vi "Untitled 1.vi"() -> ()   [LabVIEW 2015]
uses:
  <vilib>/MakerHub/LINX/Public/Peripherals/Analog/Analog Read 1 Chan.vi
  <vilib>/MakerHub/LINX/Private/Local IO/LinxI2cWrite.vi
  <vilib>/MakerHub/LINX/Public/Utilities/Check Channel.vi
  <vilib>/MakerHub/LINX/Public/Peripherals/Analog/Analog Read N Chans.vi
  <vilib>/MakerHub/LINX/Private/Local IO/LinxAnalogRead.vi
  <vilib>/MakerHub/LINX/Public/Utilities/Open Serial.vi
  <vilib>/MakerHub/LINX/Private/Utilties/Generate Error.vi
  <vilib>/MakerHub/LINX/LMH-LINX.lvlib
panel:
  in  "DAC Output Voltage":sgl min=0 max=5 step=0.001
  in  "stop":bool
  out "Voltage 2":dbl
  out "Voltage":dbl
  in  "LED":refnum<visa-resource-name>="N/A"
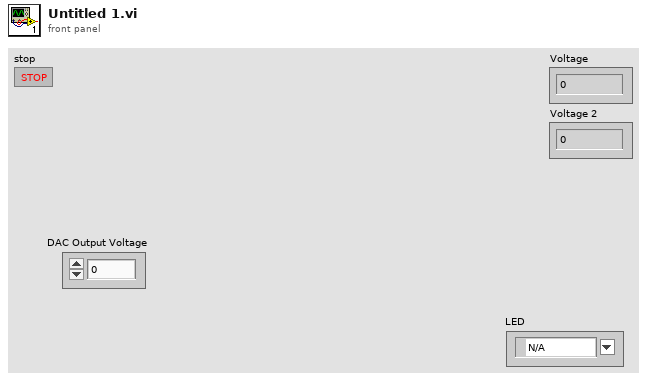
[diagram p1: front panel]
types:
  T1 = typedef "LMH-LINX.lvlib/LINX Ref.ctl" = cluster{"IO":T2, "Interface":T3, "LINX Device Config":T4}
  T2 = typedef "LMH-LINX.lvlib/Platform.ctl" = enum16{"Remote", "Local"}
  T3 = typedef "LMH-LINX.lvlib/Interface.ctl" = enum16{"Serial", "TCP"}
  T4 = typedef "LMH-LINX.lvlib/Device.lvlib/LINX Device Config.ctl" = cluster{"Interface":T3, "COM Port":refnum<visa-resource-name>, "TCP Configuration":T5, "Device Family":u8, "Device ID":u8, "Device Name":string, "TCP Ref":refnum<k5>, "Channels":T6}
  T5 = typedef "LMH-LINX.lvlib/Device.lvlib/TCP Config.ctl" = cluster{"IP Address":string, "Port":u16}
  T6 = typedef "LMH-LINX.lvlib/Channels.ctl" = cluster{"DI":u8[], "DO":u8[], "AI":u8[], "AO":u8[], "PWM":u8[], "QE":u8[], "UART":u8[], "I2C 2":u8[], "SPI":u8[], "CAN":u8[], "Servo":u8[], "AI Ref (V)":dbl, "AI Resolution (Bits)":u8, "AO Ref (V)":dbl, "AO Resolution (Bits)":u8}
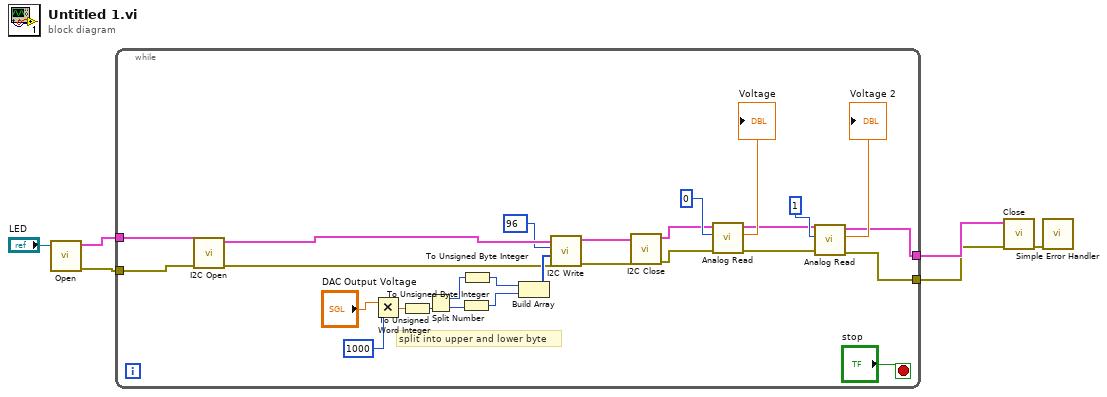
[diagram p0: block diagram]
diagram:
  n1 = call-poly <vilib>:"Open.vi"("Serial Port"="LED") -> ("Error Out"=w1:errorcluster, "LINX Resource"=w2:T1)  [unwired: 8 in, 1 out]
  n2 = while {
    tunnel: [w28] -> w4
    tunnel: [w27] -> w3
    tunnel: w2 -> [w22]
    tunnel: w1 -> [w21]
    stop <- "stop" stop-if-true
    # "split into upper and lower byte"
    n3 = call <vilib>:"I2C Open.vi"("Error In"=w21, "LINX Resource"=w22) -> ("Error Out"=w8:errorcluster, "LINX Resource"=w9:T1)  [unwired: 8 in]
    n4 = Multiply(x="DAC Output Voltage", y=u32 1000) -> (x*y=w14:sgl)
    n5 = To Unsigned Word Integer(number=w14) -> (unsigned 16bit integer=w15:u16)
    n6 = Split Number(x=w15) -> (hi(x)=w16:u8, lo(x)=w19:u8)
    n7 = To Unsigned Byte Integer(number=w19) -> (unsigned 8bit integer=w17:u8)
    n8 = To Unsigned Byte Integer(number=w16) -> (unsigned 8bit integer=w18:u8)
    n9 = Build Array(w18, w17) -> (w12:u8[])
    n10 = call <vilib>:"I2C Write.vi"("Error In"=w8, "Data"=w12, "I2C Slave Address (0)"=u8 96, "LINX Resource"=w9) -> ("Error Out"=w10:errorcluster, "LINX Resource"=w11:T1)  [unwired: 6 in]
    n11 = call <vilib>:"I2C Close.vi"("Error In"=w10, "LINX Resource"=w11) -> ("Error Out"=w23:errorcluster, "LINX Resource"=w24:T1)  [unwired: 8 in]
    n12 = call-poly <vilib>:"Analog Read.vi"("Error In"=w23, "Analog Channel"=u8 0, "LINX Resource"=w24) -> ("Error Out"=w31:errorcluster, "Voltage"=→"Voltage":dbl, "LINX Resource"=w26:T1)  [unwired: 5 in, 1 out]
    n13 = call-poly <vilib>:"Analog Read.vi"("Error In"=w31, "Analog Channel"=u8 1, "LINX Resource"=w26) -> ("Error Out"=w27:errorcluster, "Voltage"=→"Voltage 2":dbl, "LINX Resource"=w28:T1)  [unwired: 5 in, 1 out]
  }
  n14 = call <vilib>:"Close.vi"("Error In"=w3, "LINX Resource"=w4) -> ("Error Out"=w5:errorcluster)  [unwired: 9 in]
  n15 = call <vilib>:"Simple Error Handler.vi"("error in (no error)"=w5) -> ()  [unwired: 4 in, 5 out]
